vi "List Videos.vi"() -> ()   [LabVIEW 2014]
panel:
  out "filenames":string[](array[string])
  out "Listbox":i32(listbox)
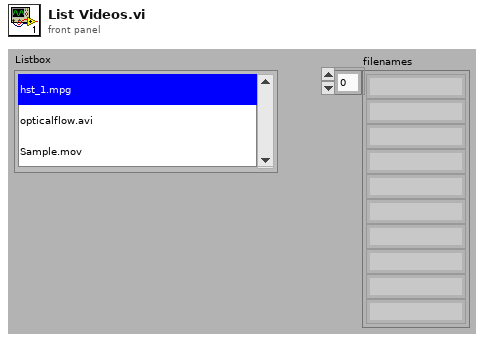
[diagram p1: front panel]
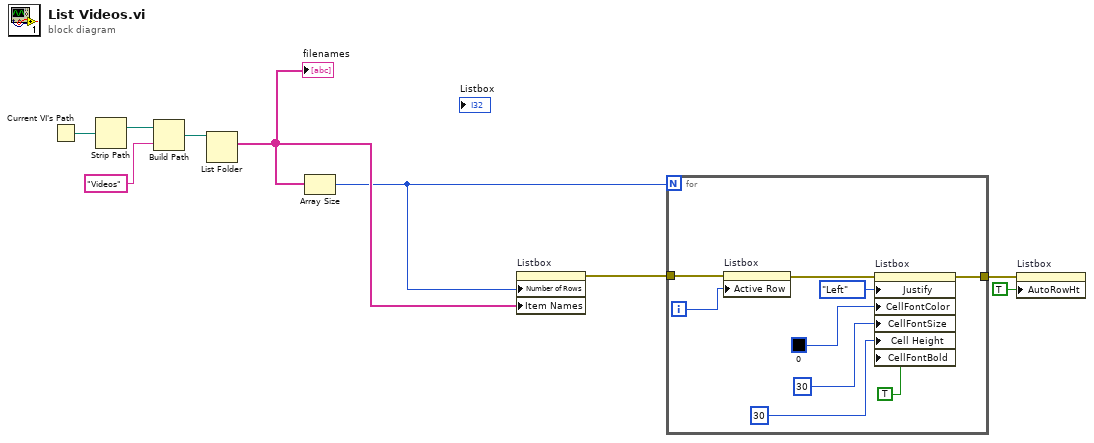
[diagram p0: block diagram]
diagram:
  n1 = Current VI's Path() -> (path=w9:path)
  n2 = Strip Path(path=w9) -> (stripped path=w8:path)  [unwired: 1 out]
  n3 = Build Path(base path=w8, name or relative path="Videos") -> (appended path=w6:path)
  n4 = List Folder(path=w6) -> (filenames=w5:string[])  [unwired: 3 in, 3 out]
  "filenames" <- w5
  n5 = Array Size(array=w5) -> (size(s)=w3:i32)
  n6 = property on="Listbox" class="LstBox (strict)"("Number of Rows"=w3, "Item Names"=w5) -> (error out=w4:errorcluster)  [unwired: 2 in, 1 out]
  n7 = for {
    N: w3 -> [_]
    tunnel: w4 -> [w18]
    tunnel: [w11] -> w2
    i -> [w12]
    n8 = property on="Listbox" class="LstBox (strict)"(error in=w18, "Active Row"=w12) -> (error out=w17:errorcluster)  [unwired: 1 in, 1 out]
    n9 = property on="Listbox" class="LstBox (strict)"(error in=w17, "Justify"=enum16{"Left", "Center", "Right"}."Left" ("Active Row:Cell Justification"), "CellFontColor"=u32 0 ("Active Row:Cell Font:Color"), "CellFontSize"=u32 30 ("Active Row:Cell Font:Size"), "Cell Height"=30 ("Active Row:Cell Height"), "CellFontBold"=TRUE ("Active Row:Cell Font:Bold")) -> (error out=w11:errorcluster)  [unwired: 1 in, 1 out]
  }
  n10 = property on="Listbox" class="LstBox (strict)"(error in=w2, "AutoRowHt"=TRUE ("Autosizing Row Height")) -> ()  [unwired: 1 in, 2 out]
